vi "Receive Shortcut Menu Selection Event.vi"(8 "error in (no error)":errorcluster, 10 "ShortcutMenuSelectionMsg":refnum<class "ShortcutMenuSelectionMsg.lvclass">, 11 "TreeActor In":refnum<class "TreeActor.lvclass">) -> (0 "error out":errorcluster, 3 "TreeActor Out":refnum<class "TreeActor.lvclass">)   [LabVIEW 2017, in "Integration Test Launcher.lvlib" / "TestViewables.lvlib" / "TreeActor.lvclass"]
doc: "<License>\nCopyright © 2020 Tymphany, LLC | All rights reserved\nwww.Tymphany.com\nHuijun <Huijun.Guo@Tymphany.com>\n</License>"
uses:
  <vilib>/gpm_packages/@cs/example/Integration Test/TreeActor/TreeActor.lvclass
  <vilib>/gpm_packages/@cs/mva-viewable/Source/ActorEvents/IEventAggregator Messages/ShortcutMenuSelectionMsg/ShortcutMenuSelectionMsg.lvclass
  <vilib>/gpm_packages/@cs/mva-viewable/Source/ActorEvents/IEventAggregator Messages/ShortcutMenuSelectionMsg/Accessors/Read Item Tag.vi
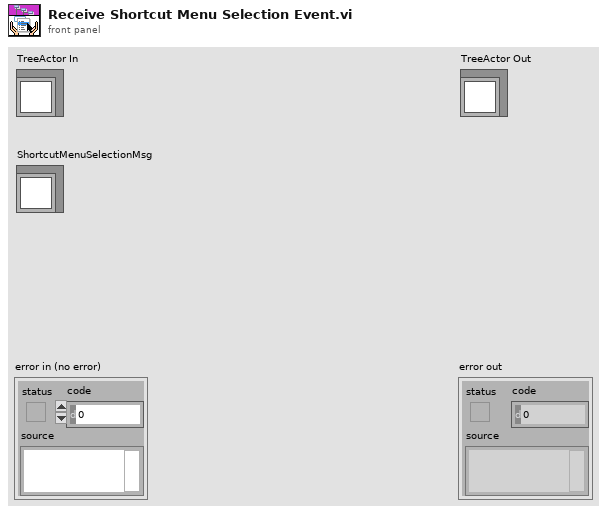
[diagram p1: front panel]
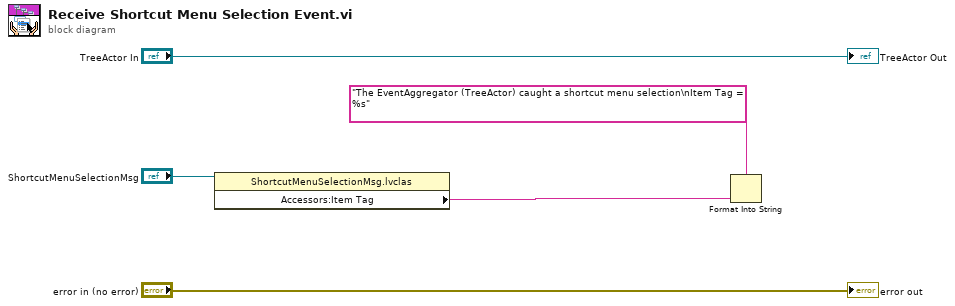
[diagram p0: block diagram]
diagram:
  n1 = property class="ShortcutMenuSelectionMsg.lvclas"(reference="ShortcutMenuSelectionMsg") -> ("Accessors:Item Tag"=w1:string)  [unwired: 1 in, 2 out]
  n2 = Format Into String(format string="The EventAggregator (TreeActor) caught a shortcut menu selection\nItem Tag = %s", w1) -> ()  [unwired: 2 in, 2 out]
  "error out" <- "error in (no error)"
  "TreeActor Out" <- "TreeActor In"
